vi "Start Intro.vi"(8 "error in":errorcluster, 9 "Saving":bool, 10 "Interface Ref":T1) -> (0 "error out":errorcluster, 2 "Ref Out":T2)   [LabVIEW 2015]
uses:
  <vilib>/myRIO/Instrument Drivers/Onboard IO/AudioOut Block/typedefs/AudioOut Block Reference.ctl
  <vilib>/myRIO/Common/Instrument Driver Framework/Utilities/typedefs/myRIO Generic Hardware Reference.ctl
  <vilib>/myRIO/Common/Instrument Driver Framework/Utilities/typedefs/Hardware Version Enum.ctl
  <vilib>/myRIO/Common/Instrument Driver Framework/Utilities/typedefs/myRIO v1.0 Reference.ctl
  <vilib>/myRIO/Common/Instrument Driver Framework/Utilities/typedefs/Generic FPGA Reference.ctl
  <vilib>/myRIO/Common/Instrument Driver Framework/myRIO v1.0/AudioOut Block/typedefs/AudioOut Block Channels List.ctl
  <vilib>/myRIO/Common/Instrument Driver Framework/myRIO v1.0/AudioOut Block/typedefs/AudioOut Block Channels Enum.ctl
  <vilib>/myRIO/Common/Instrument Driver Framework/Utilities/typedefs/Analog Scaling Constants.ctl
  TypeDefs Host/FPGA Dynamic Interface.ctl
  TypeDefs Host/Open Audio FGV Enum.ctl
  <vilib>/FPGAPlugInAG/Dynamic/niLvFpga_Close_Dynamic.vi
  <vilib>/rvi/interface/nirviCloseFPGA/nirviCloseFPGA.xnode
  <vilib>/myRIO/Instrument Drivers/Onboard IO/AudioOut Block/AudioOut Block.lvlib
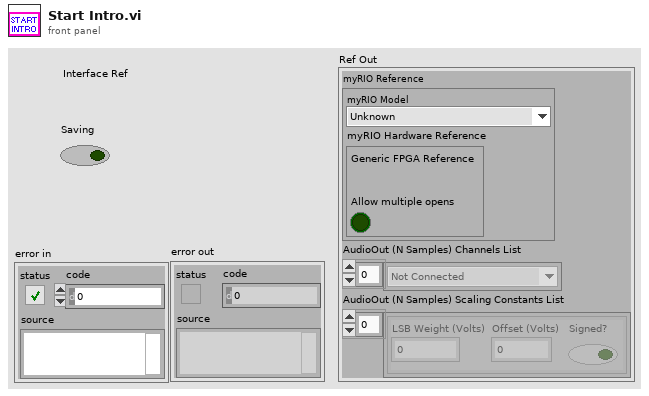
[diagram p1: front panel]
types:
  T1 = typedef "FPGA Dynamic Interface.ctl" = refnum<k20>
  T2 = typedef "AudioOut Block.lvlib/AudioOut Block Reference.ctl" = cluster{"myRIO Reference":T3, "AudioOut (N Samples) Channels List":T7, "AudioOut (N Samples) Scaling Constants List":T9[]}
  T3 = typedef "myRIO Generic Hardware Reference.ctl" = cluster{"myRIO Model":T4, "myRIO Hardware Reference":T5}
  T4 = typedef "Hardware Version Enum.ctl" = enum16{"Unknown", "myRIO-1900", "myRIO-1950", "roboRIO"}
  T5 = typedef "myRIO v1.0 Reference.ctl" = cluster{"Generic FPGA Reference":T6, "Allow multiple opens":bool}
  T6 = typedef "Generic FPGA Reference.ctl" = refnum<k20>
  T7 = typedef "AudioOut Block Channels List.ctl" = T8[]
  T8 = typedef "AudioOut Block Channels Enum.ctl" = enum16{"Not Connected", "AudioOut/Left (N Samples)", "AudioOut/Right (N Samples)"}
  T9 = typedef "Analog Scaling Constants.ctl" = cluster{"LSB Weight (Volts)":dbl, "Offset (Volts)":dbl, "Signed?":bool}
  T10 = typedef "Open Audio FGV Enum.ctl" = enum16{"Get", "Set"}
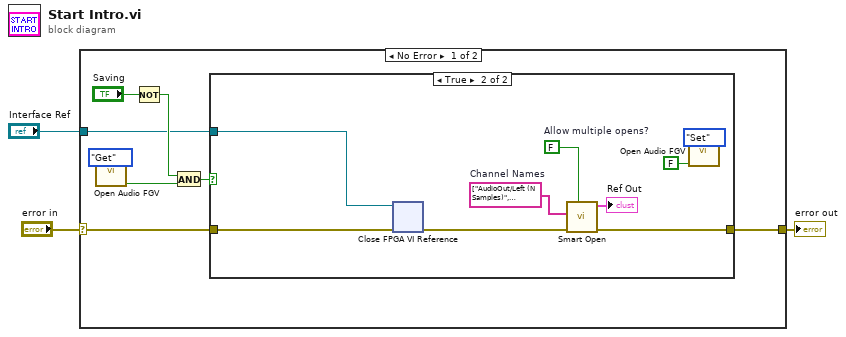
[diagram p0: block diagram]
diagram:
  n1 = case shown="No Error" "error in" {
    selector: "error in" -> [w10 w22]
    tunnel: [w11 w22] -> w3
    tunnel: "Interface Ref" -> [w4 _]
    frame No Error {
      n2 = call "Open Audio FGV.vi"("Command"=Open_Audio_FGV_Enum."Get") -> ("Open"=w8:bool)  [unwired: 10 in]
      n3 = Not(x="Saving") -> (.not. x?=w5:bool)
      n4 = And(x=w5, y=w8) -> (x .and. y?=w7:bool)
      n5 = case shown="True" w7 {
        tunnel: [w12 w18] -> w11
        tunnel: w10 -> [w12 w15]
        tunnel: w4 -> [_ w13]
        frame False {
        }
        frame True {
          w21 = tag[] ["AudioOut/Left (N Samples)", "AudioOut/Right (N Samples)"]  # Channel Names
          w20 = FALSE  # Allow multiple opens?
          n6 = xnode "Close FPGA VI Reference"("FPGA VI Reference In"=w13, "error in"=w15) -> ("error out"=w14:errorcluster)
          n7 = call <vilib>:"Smart Open.vi"("Allow multiple opens?"=w20, "error in (no error)"=w14, "Channel Names"=w21) -> ("error out"=w18:errorcluster, "AudioOut (N Samples) Ref Out"=→"Ref Out":T2)  [unwired: 7 in]
          n8 = call "Open Audio FGV.vi"("Command"=Open_Audio_FGV_Enum."Set", "Open?"=FALSE) -> ()  [unwired: 9 in, 1 out]
        }
      }
    }
    frame Error {
    }
  }
  "error out" <- w3
